vi "example.vi"() -> ()   [LabVIEW 2023]
uses:
  gfitsio.lvlib
  <vilib>/picture/picture.llb/Draw True-Color Pixmap.vi
  gfitsio-read-image-subset-i32-2d.vi
  cfitsio-bitpix.ctl
  gfitsio-write-image-subset-i32-2d.vi
panel:
  out "hdu name (dialog if empty)":string
  out "hdu names":string[](array[string])
  out "hdu name":string
  in  "Tab Control":enum32{"Complete Image", "Red", "Green", "Blue"}(tab)
  out "Complete Image":picture
  out "Red":picture
  out "Green":picture
  out "Blue":picture
  # "Run the VI to create a FITS file from a BMP image stored on disk and then read back the FITS file to populate the image below."
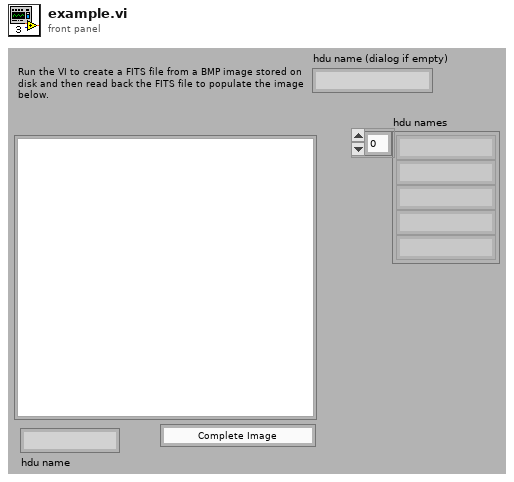
[diagram p1: front panel]
types:
  T1 = enum16{"open", "open or create", "create", "create or replace"}
  T2 = enum16{"open", "open or create", "create or replace", "create", "open (read only)"}
  T3 = typedef "gfitsio.lvlib/cfitsio-bitpix.ctl" = i32
  T4 = typedef "imagedata.ctl" = cluster{"image type":i32, "image depth":i32, "image":u8[], "mask":u8[], "colors":u32[], "Rectangle":cluster{"left":i16, "top":i16, "right":i16, "bottom":i16}}
  T5 = typedef "gfitsio.lvlib/gfitsio-refnum.ctl" = refnum<k1>
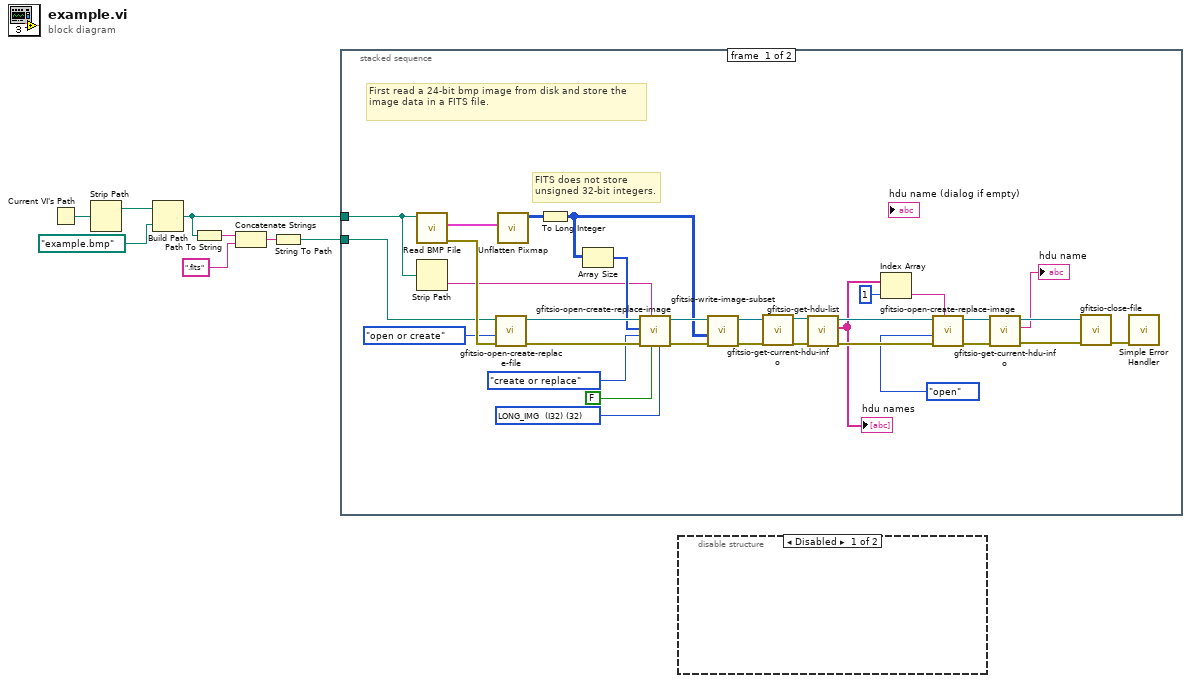
[diagram p0: block diagram]
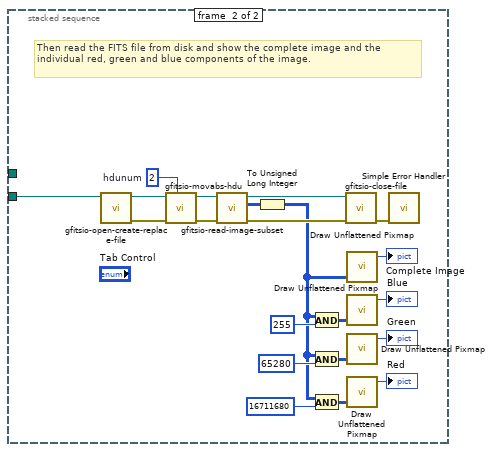
[diagram p3: hidden frame]
diagram:
  n1 = Current VI's Path() -> (path=w6:path)
  n2 = Strip Path(path=w6) -> (stripped path=w7:path)  [unwired: 1 out]
  n3 = Build Path(base path=w7, name or relative path=path "example.bmp" ("path to BMP file")) -> (appended path=w2:path)
  n4 = Path To String(path=w2) -> (string=w3:string)
  n5 = Concatenate Strings(w3, ".fits" ("string")) -> (w5:string)
  n6 = String To Path(string=w5) -> (path=w1:path)
  n7 = stacked-sequence {
    tunnel: w2 -> [w25 _]
    tunnel: w1 -> [w26 w41]
    frame #0 {
      w30 = T3 32 items=["<invalid type>"=0, "BYTE_IMG  (U8)"=8, "SHORT_IMG  (I16)"=16, "USHORT_IMG  (U16)"=20, "LONG_IMG  (I32)"=32, "ULONG_IMG  (U32)"=40, "FLOAT_IMG  (SGL)"=-32, "DOUBLE_IMG  (DBL)"=-64] ("image data type")
      # "First read a 24-bit bmp image from disk and store the image data in a FITS file."
      # "FITS does not store unsigned 32-bit integers."
      n8 = call <vilib>:"Read BMP File.vi"("path to BMP file"=w25) -> ("error out"=w36:errorcluster, "image data"=w29:T4)  [unwired: 8 in, 1 out]
      n9 = Strip Path(path=w25) -> (name=w24:string)  [unwired: 1 out]
      n10 = call "gfitsio-open-create-replace-file.vi"("error in (no error)"=w36, "function (open)"=T2."open or create", "file path (dialog if empty)"=w26) -> ("error out"=w39:errorcluster, "gfits refnum"=w40:T5)  [unwired: 6 in, 1 out]
      n11 = call <vilib>:"Unflatten Pixmap.vi"("image data"=w29) -> ("24-bit pixmap"=w35:u32[][])  [unwired: 4 in, 6 out]
      n12 = To Long Integer(number=w35) -> (32bit integer=w32:i32[][])
      n13 = Array Size(array=w32) -> (size(s)=w31:i32[])
      n14 = call "gfitsio-open-create-replace-image.vi"("image data type"=w30, "advisory dialog? (display:T)"=FALSE, "hdu name (dialog if empty)"=w24, "error in (no error)"=w39, "function (create or replace)"=T1."create or replace" ("function (open or create)"), "naxes"=w31, "gfits refnum"=w40) -> ("error out"=w38:errorcluster, "dup gfits refnum"=w37:T5)  [unwired: 2 in, 1 out]
      n15 = call-poly "gfitsio-write-image-subset.vi"("error in (no error)"=w38, "data"=w32, "gfits refnum"=w37) -> ("error out"=w22:errorcluster, "dup gfits refnum"=w23:T5)  [unwired: 7 in]
      n16 = call "gfitsio-get-current-hdu-info.vi"("error in (no error)"=w22, "gfits refnum"=w23) -> ("error out"=w20:errorcluster, "dup gfits refnum"=w21:T5)  [unwired: 5 in, 3 out]
      n17 = call "gfitsio-get-hdu-list.vi"("error in (no error)"=w20, "gfits refnum"=w21) -> ("error out"=w18:errorcluster, "hdu names"=w11:string[], "dup gfits refnum"=w19:T5)  [unwired: 6 in, 1 out]
      "hdu names" <- w11
      n18 = Index Array(array=w11, index=1) -> (element=w10:string)
      n19 = call "gfitsio-open-create-replace-image.vi"("hdu name (dialog if empty)"=w10, "error in (no error)"=w18, "function (create or replace)"=T1."open", "gfits refnum"=w19) -> ("error out"=w15:errorcluster, "dup gfits refnum"=w16:T5)  [unwired: 5 in, 1 out]
      n20 = call "gfitsio-get-current-hdu-info.vi"("error in (no error)"=w15, "gfits refnum"=w16) -> ("error out"=w13:errorcluster, "hdu name"=→"hdu name":string, "dup gfits refnum"=w14:T5)  [unwired: 5 in, 2 out]
      n21 = call "gfitsio-close-file.vi"("error in (no error)"=w13, "gfits refnum"=w14) -> ("error out"=w28:errorcluster)  [unwired: 8 in, 1 out]
      n22 = call <vilib>:"Simple Error Handler.vi"("error in (no error)"=w28) -> ()  [unwired: 4 in, 5 out]
    }
    frame #1 {
      w54 = 2  # hdunum
      # "Then read the FITS file from disk and show the complete image and the individual red, green and blue components of the image."
      n23 = call "gfitsio-open-create-replace-file.vi"("file path (dialog if empty)"=w41) -> ("error out"=w61:errorcluster, "gfits refnum"=w60:T5)  [unwired: 8 in, 1 out]
      n24 = call "gfitsio-movabs-hdu.vi"("hdunum"=w54, "error in (no error)"=w61, "gfits refnum"=w60) -> ("error out"=w59:errorcluster, "dup gfits refnum"=w58:T5)  [unwired: 6 in, 1 out]
      n25 = call-poly "gfitsio-read-image-subset.vi"("error in (no error)"=w59, "gfits refnum"=w58) -> ("error out"=w57:errorcluster, "data"=w53:i32[][], "dup gfits refnum"=w56:T5)  [unwired: 7 in]
      n26 = To Unsigned Long Integer(number=w53) -> (unsigned 32bit integer=w42:u32[][])
      n27 = And(x=w42, y=u32 255) -> (x .and. y?=w49:u32[][])
      n28 = And(x=w42, y=u32 65280) -> (x .and. y?=w46:u32[][])
      n29 = And(x=w42, y=u32 16711680) -> (x .and. y?=w44:u32[][])
      n30 = call "gfitsio-close-file.vi"("error in (no error)"=w57, "gfits refnum"=w56) -> ("error out"=w55:errorcluster)  [unwired: 8 in, 1 out]
      n31 = call-poly <vilib>:"Draw Unflattened Pixmap.vi"("data (RGB format)"=w42) -> ("new picture"=→"Complete Image":picture)  [unwired: 8 in]
      n32 = call-poly <vilib>:"Draw Unflattened Pixmap.vi"("data (RGB format)"=w49) -> ("new picture"=→"Blue":picture)  [unwired: 8 in]
      n33 = call-poly <vilib>:"Draw Unflattened Pixmap.vi"("data (RGB format)"=w46) -> ("new picture"=→"Green":picture)  [unwired: 8 in]
      n34 = call-poly <vilib>:"Draw Unflattened Pixmap.vi"("data (RGB format)"=w44) -> ("new picture"=→"Red":picture)  [unwired: 8 in]
      n35 = call <vilib>:"Simple Error Handler.vi"("error in (no error)"=w55) -> ()  [unwired: 4 in, 5 out]
    }
  }
  n36 = disable-structure shown="Disabled" {
    frame Disabled {
    }
    frame Enabled {
    }
  }
